vi "test_ClientFGV_GetClientThenRecreateClient_ClientCreatedTwice.vi"(8 "error in":errorcluster) -> (0 "error out":errorcluster, 2 "result":string, 3 "pass":bool)   [LabVIEW 2020, in "MeasurementServerTests.lvlib" / "gRPC Utilities Tests.lvlib"]
uses:
  gRPC Utilities Tests.lvlib
  Runtime/MeasurementLink gRPC Utilities/gRPC Client Pool Helpers/Action.ctl
  Runtime/MeasurementLink gRPC Utilities/MeasurementLink gRPC Utilities.lvlib
  <vilib>/gRPC/LabVIEW gRPC Library/Shared/grpcId.ctl
  <vilib>/gRPC/LabVIEW gRPC Library/grpc-lvsupport-release.lvlib
  Action.ctl
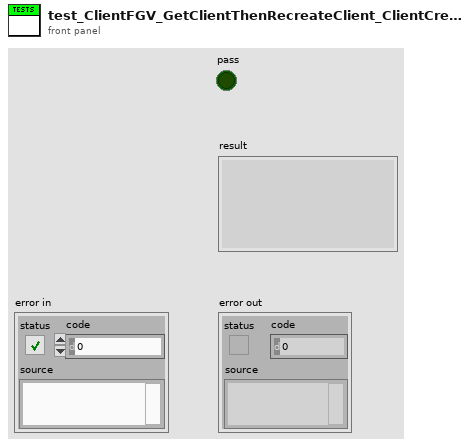
[diagram p1: front panel]
types:
  T1 = typedef "Action.ctl" = enum16{"Increment Id", "Reset", "Error on Next Call"}
  T2 = typedef "grpc-lvsupport-release.lvlib/grpcId.ctl" = u64
  T3 = typedef "MeasurementLink gRPC Utilities.lvlib/Action.ctl" = enum16{"Get Client", "Recreate Client"}
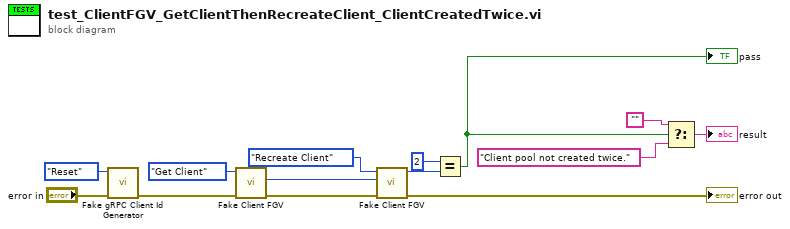
[diagram p0: block diagram]
diagram:
  n1 = call "Fake gRPC Client Id Generator.vi"("error in"="error in", "action"=Action."Reset") -> ("error out"=w6:errorcluster)  [unwired: 8 in, 1 out]
  n2 = call "Fake Client FGV.vi"("error in"=w6, "action"=Action."Get Client") -> ("error out"=w8:errorcluster, "unique id out"=w2:u64)  [unwired: 7 in, 1 out]
  n3 = call "Fake Client FGV.vi"("error in"=w8, "unique id in"=w2, "action"=Action."Recreate Client") -> ("error out"=→"error out":errorcluster, "grpc client id"=w5:T2)  [unwired: 6 in, 1 out]
  n4 = Equal?(x=T2 2, y=w5) -> (x = y?=w3:bool)
  "pass" <- w3
  n5 = Select(t="", s=w3, f="Client pool not created twice.") -> (s? t:f=→"result":string)
